vi "cube vision.vi"() -> ()   [LabVIEW 2017]
uses:
  <vilib>/vision/NI_Vision_Development_Module.lvlib
panel:
  in  "scale":i32=2
  out "angle":dbl
  out "Color":T1(plugin-control)
  out "Binary Image":T1(plugin-control)
  in  "Sat Range":cluster{u8, u8}(slide)={255, 120} scale=0.0..255.0
  in  "Hue Range":cluster{u8, u8}(slide)={207, 119} scale=0.0..255.0
  in  "File Path":path=path "C:/Users/19LES01/Documents/LabView/2017/vision/3792_Vision_2017/high goal 320x240.bmp"
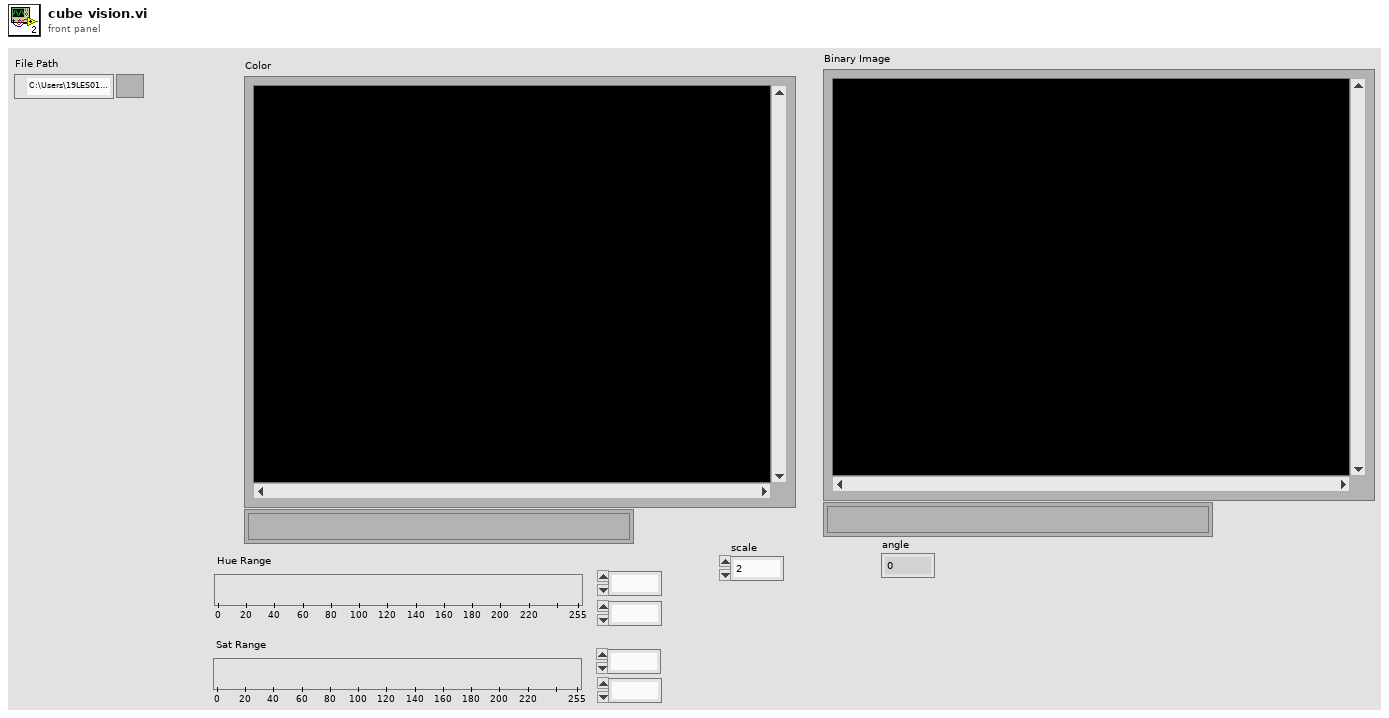
[diagram p1: front panel]
types:
  T1 = typedef "IMAQ Image.ctl" = refnum<image>
  T2 = typedef "Image Type" = u32
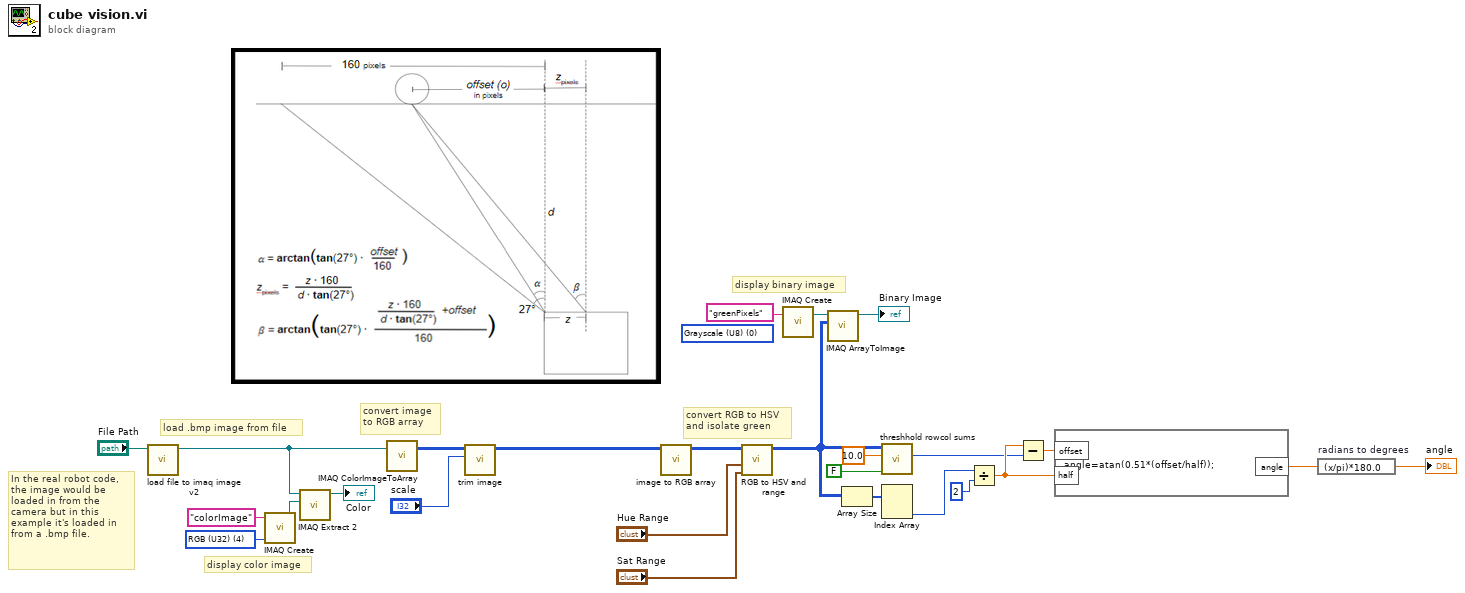
[diagram p0: block diagram]
diagram:
  (unwired) T2 0 items=["Grayscale (U8)", "Grayscale (I16)", "Grayscale (SGL)", "Complex (CSG)", "RGB (U32)", "HSL (U32)", "RGB (U64)", "Grayscale (U16)"] ("Image Type")
  w24 = T2 4 items=["Grayscale (U8)", "Grayscale (I16)", "Grayscale (SGL)", "Complex (CSG)", "RGB (U32)", "HSL (U32)", "RGB (U64)", "Grayscale (U16)"] ("Image Type")
  # "display binary image"
  # "In the real robot code, the image would be loaded in from the camera but in this example it's loaded in from a .bmp file."
  # "convert image\nto RGB array"
  # "display color image"
  # "load .bmp image from file"
  # "convert RGB to HSV\nand isolate green"
  n1 = call "load file to imaq image v2.vi"("path to BMP file"="File Path") -> ("Image"=w17:T1)  [unwired: 9 in, 1 out]
  n2 = call "IMAQ Create"("Image Name"="colorImage", "Image Type"=w24) -> ("New Image"=w26:T1)  [unwired: 3 in, 1 out]
  n3 = call "IMAQ Extract 2"("Image Dst"=w26, "Image Src"=w17) -> ("Image Dst Out"=→"Color":T1)  [unwired: 8 in, 1 out]
  n4 = call "IMAQ ColorImageToArray"("Image"=w17) -> ("Image Pixels (U32)"=w3:u32[][])  [unwired: 3 in, 2 out]
  n5 = call "trim image.vi"("scale"="scale", "Image Pixels (U32)"=w3) -> ("Trimmed Image Pixels (U32)"=w2:u32[][])  [unwired: 9 in]
  n6 = call "image to RGB array.vi"("Image Pixels (U32)"=w2) -> ("Image Pixels (U8)"=w22:u8[][][])  [unwired: 10 in]
  n7 = call "RGB to HSV and range.vi"("Image Pixels (RGB)"=w22, "Hue Range"="Hue Range", "Sat Range"="Sat Range") -> ("Threshholded Pixels"=w11:u8[][])  [unwired: 7 in]
  n8 = call "IMAQ Create"("Image Name"="greenPixels") -> ("New Image"=w18:T1)  [unwired: 4 in, 1 out]
  n9 = call "IMAQ ArrayToImage"("Image Pixels (U8)"=w11, "Image"=w18) -> ("Image Out"=→"Binary Image":T1)  [unwired: 8 in, 1 out]
  n10 = Array Size(array=w11) -> (size(s)=w12:i32[])
  n11 = call "threshhold rowcol sums.vi"("Row(T)/Col(F)"=FALSE, "Threshold"=10.0, "Pixels"=w11) -> ("middle row/col"=w5:i32)  [unwired: 6 in, 2 out]
  n12 = Index Array(array=w12) -> (element #2=w1:i32)  [unwired: 2 in, 1 out]
  n13 = Divide(x=w1, y=2) -> (x/y=w6:dbl)
  n14 = Subtract(x=w6, y=w5) -> (x-y=w7:dbl)
  n15 = formula code="angle=atan(0.51*(offset/half));"("offset"=w7, "half"=w6) -> ("angle"=w9:dbl)
  n16 = expression code="(x/pi)*180.0" "radians to degrees"(w9) -> (→"angle":dbl)
